vi "Motor Control.vi"(8 "error in (no error)":errorcluster, 9 "MotorSelect":i16, 10 "INSpeed":i16, 11 "VISA Refnum in":refnum<visa-resource-name>) -> (0 "error out":errorcluster, 3 "VISA Refnum out":refnum<visa-resource-name>)   [LabVIEW 2019]
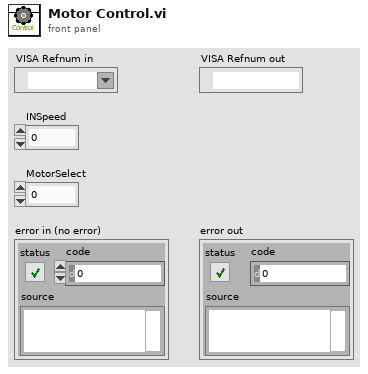
[diagram p1: front panel]
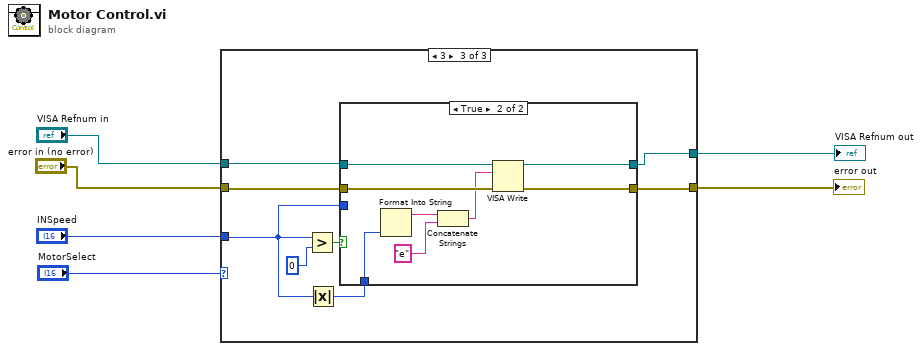
[diagram p0: block diagram]
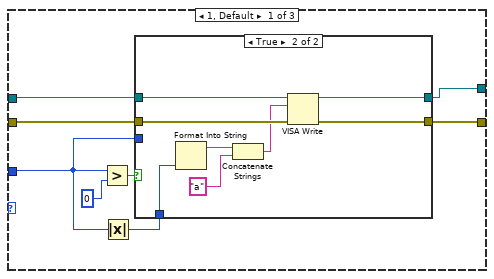
[diagram p2: hidden frame]
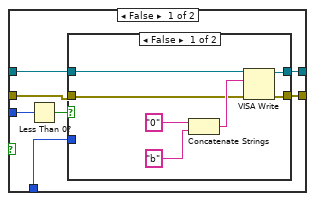
[diagram p3: hidden frame]
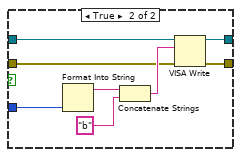
[diagram p4: hidden frame]
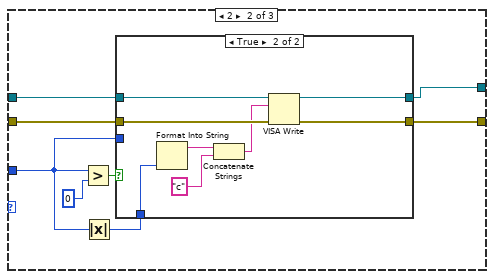
[diagram p5: hidden frame]
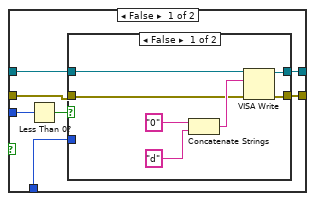
[diagram p6: hidden frame]
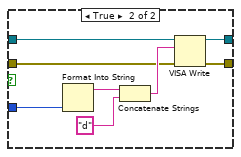
[diagram p7: hidden frame]
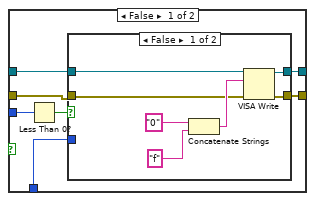
[diagram p8: hidden frame]
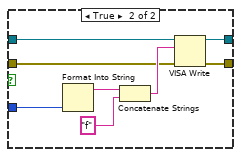
[diagram p9: hidden frame]
diagram:
  n1 = case shown="3" "MotorSelect" {
    tunnel: [w7 w52 w84] -> w1
    tunnel: "INSpeed" -> [w11 w51 w83]
    tunnel: [w8 w47 w85] -> w3
    tunnel: "VISA Refnum in" -> [w10 w46 w87]
    tunnel: "error in (no error)" -> [w9 w45 w86]
    frame 1, Default {
      n2 = Greater?(x=w11, y=i16 0) -> (0:w14:bool)
      n3 = Absolute Value(x=w11) -> (abs(x)=w13:i16)
      n4 = case shown="True" w14 {
        tunnel: w10 -> [w20 w44]
        tunnel: w9 -> [w19 w43]
        tunnel: w11 -> [w18 _]
        tunnel: [w17 w39] -> w8
        tunnel: [w16 w38] -> w7
        tunnel: w13 -> [w15 w37]
        frame False {
          n5 = Less Than 0?(x=w18) -> (x < 0?=w21:bool)
          n6 = case shown="False" w21 {
            tunnel: w20 -> [w26 w33]
            tunnel: w19 -> [w25 w32]
            tunnel: w15 -> [_ w31]
            tunnel: [w24 w30] -> w17
            tunnel: [w23 w29] -> w16
            frame False {
              n7 = Concatenate Strings("0" ("string"), "b" ("string")) -> (w28:string)
              n8 = VISA Write(VISA resource name=w26, write buffer=w28, error in (no error)=w25) -> (VISA resource name out=w24:refnum<visa-resource-name>, error out=w23:errorcluster)  [unwired: 1 out]
            }
            frame True {
              n9 = Format Into String(w31) -> (resulting string=w36:string)  [unwired: 3 in, 1 out]
              n10 = Concatenate Strings(w36, "b" ("string")) -> (w35:string)
              n11 = VISA Write(VISA resource name=w33, write buffer=w35, error in (no error)=w32) -> (VISA resource name out=w30:refnum<visa-resource-name>, error out=w29:errorcluster)  [unwired: 1 out]
            }
          }
        }
        frame True {
          n12 = Format Into String(w37) -> (resulting string=w42:string)  [unwired: 3 in, 1 out]
          n13 = Concatenate Strings(w42, "a" ("string")) -> (w40:string)
          n14 = VISA Write(VISA resource name=w44, write buffer=w40, error in (no error)=w43) -> (VISA resource name out=w39:refnum<visa-resource-name>, error out=w38:errorcluster)  [unwired: 1 out]
        }
      }
    }
    frame 2 {
      n15 = Greater?(x=w51, y=i16 0) -> (0:w49:bool)
      n16 = Absolute Value(x=w51) -> (abs(x)=w50:i16)
      n17 = case shown="True" w49 {
        tunnel: w46 -> [w58 w82]
        tunnel: w45 -> [w57 w81]
        tunnel: w51 -> [w56 _]
        tunnel: [w55 w77] -> w47
        tunnel: [w54 w76] -> w52
        tunnel: w50 -> [w53 w75]
        frame False {
          n18 = Less Than 0?(x=w56) -> (x < 0?=w59:bool)
          n19 = case shown="False" w59 {
            tunnel: w58 -> [w64 w71]
            tunnel: w57 -> [w63 w70]
            tunnel: w53 -> [_ w69]
            tunnel: [w62 w68] -> w55
            tunnel: [w61 w67] -> w54
            frame False {
              n20 = Concatenate Strings("0" ("string"), "d" ("string")) -> (w66:string)
              n21 = VISA Write(VISA resource name=w64, write buffer=w66, error in (no error)=w63) -> (VISA resource name out=w62:refnum<visa-resource-name>, error out=w61:errorcluster)  [unwired: 1 out]
            }
            frame True {
              n22 = Format Into String(w69) -> (resulting string=w74:string)  [unwired: 3 in, 1 out]
              n23 = Concatenate Strings(w74, "d" ("string")) -> (w73:string)
              n24 = VISA Write(VISA resource name=w71, write buffer=w73, error in (no error)=w70) -> (VISA resource name out=w68:refnum<visa-resource-name>, error out=w67:errorcluster)  [unwired: 1 out]
            }
          }
        }
        frame True {
          n25 = Format Into String(w75) -> (resulting string=w80:string)  [unwired: 3 in, 1 out]
          n26 = Concatenate Strings(w80, "c" ("string")) -> (w78:string)
          n27 = VISA Write(VISA resource name=w82, write buffer=w78, error in (no error)=w81) -> (VISA resource name out=w77:refnum<visa-resource-name>, error out=w76:errorcluster)  [unwired: 1 out]
        }
      }
    }
    frame 3 {
      n28 = Greater?(x=w83, y=i16 0) -> (0:w89:bool)
      n29 = Absolute Value(x=w83) -> (abs(x)=w90:i16)
      n30 = case shown="True" w89 {
        tunnel: w87 -> [w96 w120]
        tunnel: w86 -> [w95 w119]
        tunnel: w83 -> [w94 _]
        tunnel: [w93 w115] -> w85
        tunnel: [w92 w114] -> w84
        tunnel: w90 -> [w91 w113]
        frame False {
          n31 = Less Than 0?(x=w94) -> (x < 0?=w97:bool)
          n32 = case shown="False" w97 {
            tunnel: w96 -> [w102 w109]
            tunnel: w95 -> [w101 w108]
            tunnel: w91 -> [_ w107]
            tunnel: [w100 w106] -> w93
            tunnel: [w99 w105] -> w92
            frame False {
              n33 = Concatenate Strings("0" ("string"), "f" ("string")) -> (w104:string)
              n34 = VISA Write(VISA resource name=w102, write buffer=w104, error in (no error)=w101) -> (VISA resource name out=w100:refnum<visa-resource-name>, error out=w99:errorcluster)  [unwired: 1 out]
            }
            frame True {
              n35 = Format Into String(w107) -> (resulting string=w112:string)  [unwired: 3 in, 1 out]
              n36 = Concatenate Strings(w112, "f" ("string")) -> (w111:string)
              n37 = VISA Write(VISA resource name=w109, write buffer=w111, error in (no error)=w108) -> (VISA resource name out=w106:refnum<visa-resource-name>, error out=w105:errorcluster)  [unwired: 1 out]
            }
          }
        }
        frame True {
          n38 = Format Into String(w113) -> (resulting string=w118:string)  [unwired: 3 in, 1 out]
          n39 = Concatenate Strings(w118, "e" ("string")) -> (w116:string)
          n40 = VISA Write(VISA resource name=w120, write buffer=w116, error in (no error)=w119) -> (VISA resource name out=w115:refnum<visa-resource-name>, error out=w114:errorcluster)  [unwired: 1 out]
        }
      }
    }
  }
  "error out" <- w1
  "VISA Refnum out" <- w3
